vi "get control position Y.vi"(8 "error in (no error)":errorcluster, 10 "ignore caption & label? (T)":bool=TRUE, 11 "Control in":refnum<class "Control.lvclass">) -> (0 "error out":errorcluster, 3 "Control out":refnum<class "Control.lvclass">)   [LabVIEW 2010, in "Control.lvclass"]
uses:
  Control.lvclass
  Control.lvclass/Control.ctl
panel:
  out "Y":i32
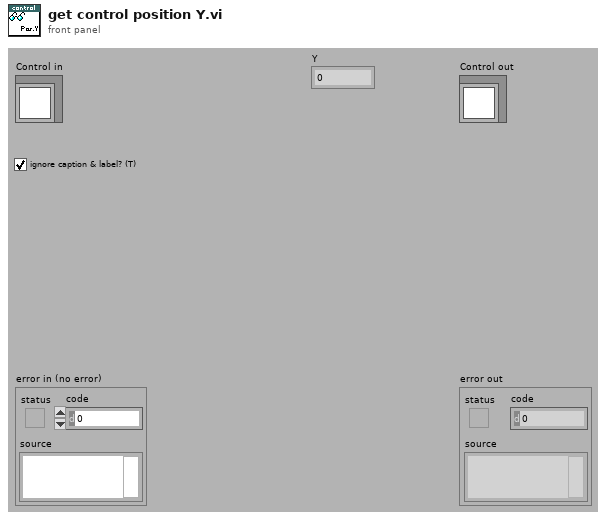
[diagram p1: front panel]
types:
  T1 = typedef "LVRectTypeDef.ctl" = cluster{"left":i16, "top":i16, "right":i16, "bottom":i16}
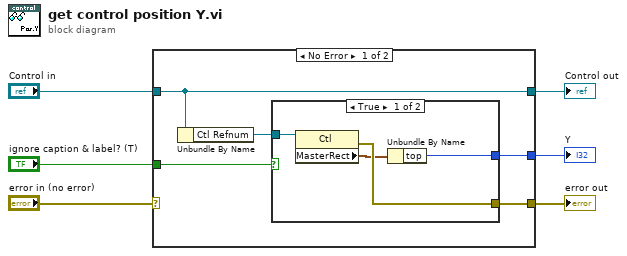
[diagram p0: block diagram]
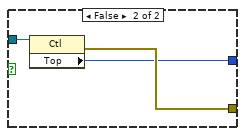
[diagram p2: hidden frame]
diagram:
  n1 = case shown="No Error" "error in (no error)" {
    selector: "error in (no error)" -> [_ w20]
    tunnel: [w9 w20] -> w5
    tunnel: [w11 w19] -> w3
    tunnel: "Control in" -> [w11 w19]
    tunnel: "ignore caption & label? (T)" -> [w8 _]
    tunnel: [w7 _] -> w1
    frame No Error {
      n2 = Unbundle By Name(w11) -> ("Ctl Refnum"=w10:refnum<vi>)
      n3 = case shown="True" w8 {
        tunnel: w10 -> [w15 w18]
        tunnel: [w14 w17] -> w9
        tunnel: [w12 w16] -> w7
        frame True {
          n4 = property class="Ctl"(reference=w15) -> (error out=w14:errorcluster, "MasterRect"=w13:T1)  [unwired: 1 in, 1 out]
          n5 = Unbundle By Name(w13) -> ("top"=w12:i16)
        }
        frame False {
          n6 = property class="Ctl"(reference=w18) -> (error out=w17:errorcluster, "Top"=w16:i32)  [unwired: 1 in, 1 out]
        }
      }
    }
    frame Error {
    }
  }
  "error out" <- w5
  "Control out" <- w3
  "Y" <- w1
